vi "generate pid channel name.vi"(10 "Channel Type":T1(ring), 11 "Identifier":string) -> (3 "Channel Name":string)   [LabVIEW 2014, in "Tagbus PID Module configuration.lvclass"]
doc: "This VI takes in a PID Loop ID and appends, the appropriate channel suffix to it, and returns the appropriate channel name."
uses:
  Tagbus PID Module configuration.lvclass
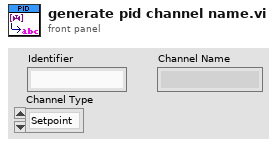
[diagram p1: front panel]
types:
  T1 = enum16{"Setpoint", "Gains", "Range", "Process Variable", "Output"}
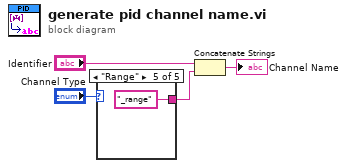
[diagram p0: block diagram]
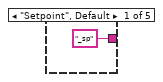
[diagram p2: hidden frame]
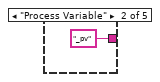
[diagram p3: hidden frame]
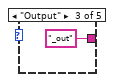
[diagram p4: hidden frame]
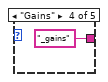
[diagram p5: hidden frame]
diagram:
  n1 = case shown="\"Range\"" "Channel Type" {
    tunnel: ["_sp" ("string") "_pv" ("string") "_out" ("string") "_gains" ("string") "_range" ("string")] -> w1
    frame "Setpoint", Default {
    }
    frame "Process Variable" {
    }
    frame "Output" {
    }
    frame "Gains" {
    }
    frame "Range" {
    }
  }
  n2 = Concatenate Strings("Identifier", w1) -> (→"Channel Name":string)
